vi "Calculate Major Scale Frequency Array.vi"(1 "# of Major Scale In":string) -> (0 "Major Scale Frequencies Out":dbl[](array[numeric]))   [LabVIEW 2020]
doc: "Calculate Major Scale Frequency Array.vi takes in the number of the major scale (0->C, etc.) the user wants to play in and outputs an array of the frequencies in that scale relative to middle X."
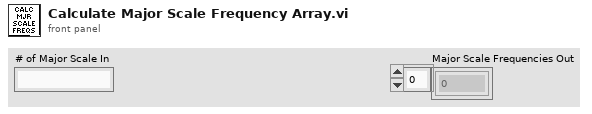
[diagram p1: front panel]
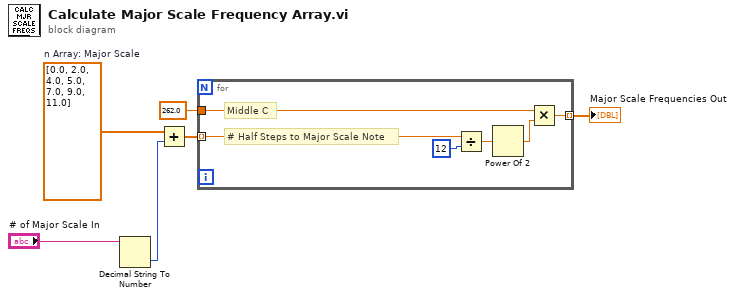
[diagram p0: block diagram]
diagram:
  w5 = dbl[] [0.0, 2.0, 4.0, 5.0, 7.0, 9.0, 11.0]  # n Array: Major Scale
  n1 = Decimal String To Number(string="# of Major Scale In") -> (number=w3:i32)  [unwired: 2 in, 1 out]
  n2 = Add(x=w5, y=w3) -> (x+y=w4:dbl[])
  n3 = for {
    tunnel: 262.0 ("x") -> [w8]
    tunnel: [w9] -> w2 mode=indexing
    tunnel: w4 -> [w7] mode=indexing
    # "Middle C"
    # "# Half Steps to Major Scale Note"
    n4 = Divide(x=w7, y=12) -> (x/y=w12:dbl)
    n5 = Power Of 2(x=w12) -> (2^x=w11:dbl)
    n6 = Multiply(x=w8, y=w11) -> (x*y=w9:dbl)
  }
  "Major Scale Frequencies Out" <- w2
